vi "Init Class Dialog.vi"(8 "error in (no error)":errorcluster, 9 "ModelRef":refnum<vi>, 10 "CategoryRef":refnum<vi>, 11 "Configuration in":refnum<class "Configuration.lvclass">) -> (0 "error out":errorcluster, 3 "Configuration out":refnum<class "Configuration.lvclass">, 5 "Base Path":path=path "C:/Users/Public/Documents/Development/builds/Instruments")   [LabVIEW 2023, in "Configuration.lvlib" / "Configuration.lvclass"]
uses:
  Library/Configuration.lvclass
  Library/Configuration.lvclass/Configuration.ctl
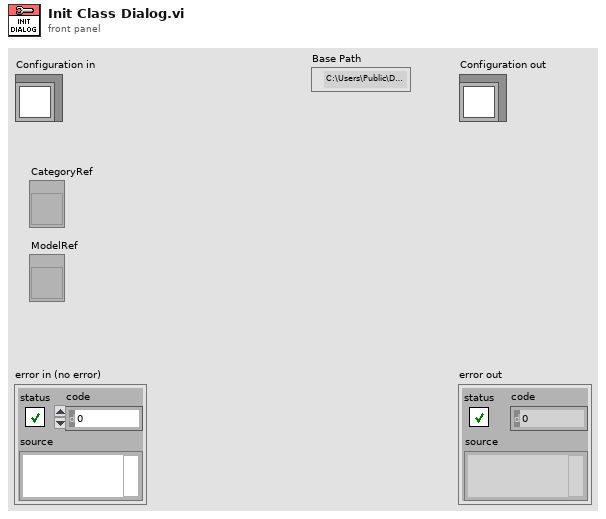
[diagram p1: front panel]
types:
  T1 = enum8{"Enabled", "Disabled", "Disabled and Grayed Out"}
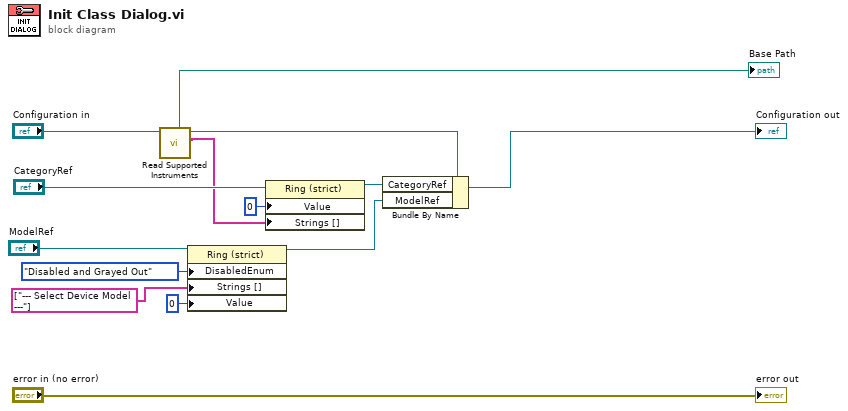
[diagram p0: block diagram]
diagram:
  n1 = call "Read Supported Instruments.vi"("Configuration in"="Configuration in") -> ("Instruments"=w1:string[], "Configuration out"=w3:refnum<class "Configuration.lvclass">, "Base Path"=→"Base Path":path)  [unwired: 7 in, 1 out]
  n2 = property class="Ring (strict)"(reference="ModelRef", "DisabledEnum"=T1."Disabled and Grayed Out" ("Disabled"), "Strings []"=string[] ["--- Select Device Model ---"], "Value"=u16 0) -> (reference out=w7:refnum<vi>)  [unwired: 1 in, 1 out]
  n3 = property class="Ring (strict)"(reference="CategoryRef", "Value"=u16 0, "Strings []"=w1) -> (reference out=w8:refnum<vi>)  [unwired: 1 in, 1 out]
  n4 = Bundle By Name(cluster=w3, "CategoryRef"=w8, "ModelRef"=w7) -> (→"Configuration out":refnum<class "Configuration.lvclass">)
  "error out" <- "error in (no error)"
